vi "create_report.vi"(8 "error in (no error)":errorcluster, 9 "prog_started":bool, 10 "Current VI Reference":refnum<vi>, 11 "TabControl in":refnum<vi>) -> (0 "error out":errorcluster, 3 "States":string)   [LabVIEW 2019]
uses:
  <vilib>/printing/ReportDocExtensions.llb/Append Front Panel Image to Report (refnum).vi
  <vilib>/Platform/browser.llb/Open URL in Default Browser (path).vi
  <vilib>/Utility/NIReport.llb/NI_report.lvclass
  <vilib>/Utility/NIReport.llb/NI_ReportGenerationCore.lvlib
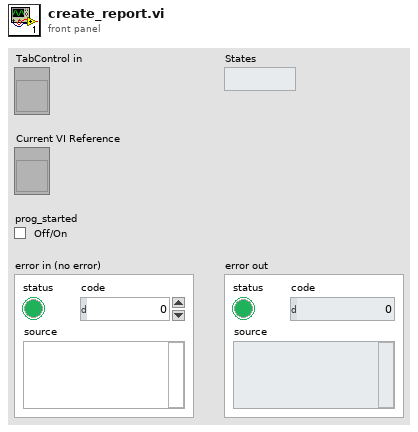
[diagram p1: front panel]
types:
  T1 = enum16{"open", "replace", "create", "open or create", "replace or create", "replace or create with confirmation"}
  T2 = enum32{"Experiment", "Resistivity ", "Seebeck", "Hardware"}
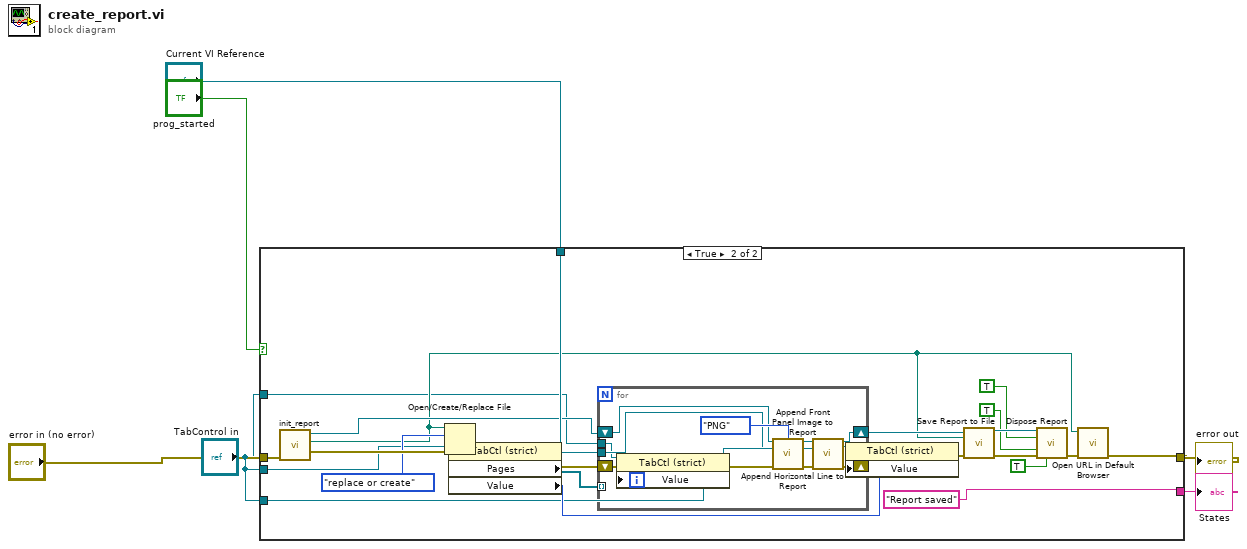
[diagram p0: block diagram]
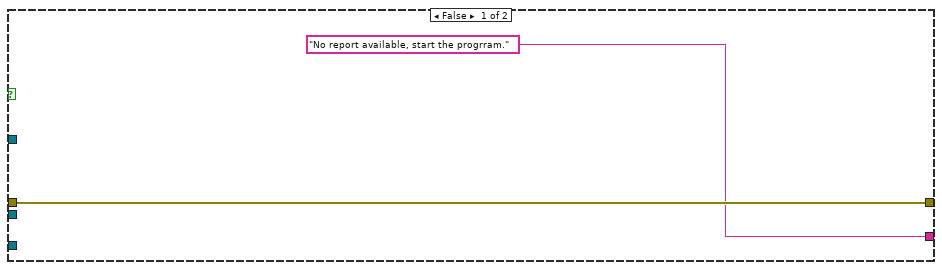
[diagram p2: hidden frame]
diagram:
  n1 = case shown="True" "prog_started" {
    tunnel: "Current VI Reference" -> [_ w32]
    tunnel: [w8 w31] -> w3
    tunnel: "error in (no error)" -> [w8 w16]
    tunnel: ["No report available, start the progrram." ("States") "Report saved" ("States")] -> w6
    tunnel: "TabControl in" -> [_ w11]
    tunnel: "TabControl in" -> [_ w10]
    tunnel: "TabControl in" -> [_ w9]
    frame False {
    }
    frame True {
      n2 = call "init_report.vi"("error in"=w16) -> ("error out"=w18:errorcluster, "appended path"=w13:path, "NI_report out"=w15:refnum<class "NI_report.lvclass">)  [unwired: 8 in]
      n3 = Open/Create/Replace File(file path (use dialog)=w13, error in=w18, operation (0:open)=T1."replace or create") -> (error out=w14:errorcluster)  [unwired: 3 in, 2 out]
      n4 = property on="Property Node" class="TabCtl (strict)"(reference=w10, error in=w14) -> (error out=w22:errorcluster, "Pages"=w23:refnum<vi>[], "Value"=w19:T2)  [unwired: 1 out]
      n5 = for {
        tunnel: w32 -> [w40]
        shift-right: [w39] -> w21
        shift-left: w22 -> [w36]
        shift-right: [w38] -> w25
        shift-left: w15 -> [w37]
        tunnel: w23 -> [_] mode=indexing
        tunnel: w11 -> [w33]
        i -> [w34]
        n6 = property on="Property Node" class="TabCtl (strict)"(reference=w33, error in=w36, "Value"=w34) -> (error out=w35:errorcluster)  [unwired: 1 out]
        n7 = call-poly <vilib>:"Append Front Panel Image to Report.vi"("report in"=w37, "image format (jpeg)"=enum32{"PNG", "JPEG", "GIF"}."PNG", "VI"=w40, "error in (no error)"=w35) -> ("report out"=w43:refnum<class "NI_report.lvclass">, "error out"=w42:errorcluster)  [unwired: 7 in, 3 out]
        n8 = call-dynamic "Append Horizontal Line to Report.vi"("report in"=w43, "error in (no error)"=w42) -> ("report out"=w38:refnum<class "NI_report.lvclass">, "error out"=w39:errorcluster)  [unwired: 12 in]
      }
      n9 = property on="Property Node" class="TabCtl (strict)"(reference=w9, error in=w21, "Value"=w19) -> (error out=w20:errorcluster)  [unwired: 1 out]
      n10 = call-dynamic "Save Report to File.vi"("report in"=w25, "report file path"=w13, "error in (no error)"=w20) -> ("report out"=w30:refnum<class "NI_report.lvclass">, "error out"=w24:errorcluster)  [unwired: 11 in]
      n11 = call-dynamic "Dispose Report.vi"("report in"=w30, "wait until printing completed? (T)"=TRUE, "save changes? (F)"=TRUE, "error in (no error)"=w24, "close report? (T)"=TRUE) -> ("error out"=w26:errorcluster)  [unwired: 10 in]
      n12 = call-poly <vilib>:"Open URL in Default Browser.vi"("error in (no error)"=w26, "path"=w13) -> ("error out"=w31:errorcluster)  [unwired: 4 in, 1 out]
    }
  }
  "States" <- w6
  "error out" <- w3
